vi "Write Standad Header Python.vi"(8 "error in (no error)":errorcluster, 11 "Save Image in":refnum<class "Save Image.lvclass">) -> (0 "error out":errorcluster, 3 "Save Image out":refnum<class "Save Image.lvclass">)   [LabVIEW 2018, in "Save Image.lvclass"]
uses:
  Save Image.lvclass
  Save Image.lvclass/Save Image.ctl
  Simulated_Header/Simulated_Header.lvclass
  Python Toolkit/Python Toolkit.lvclass
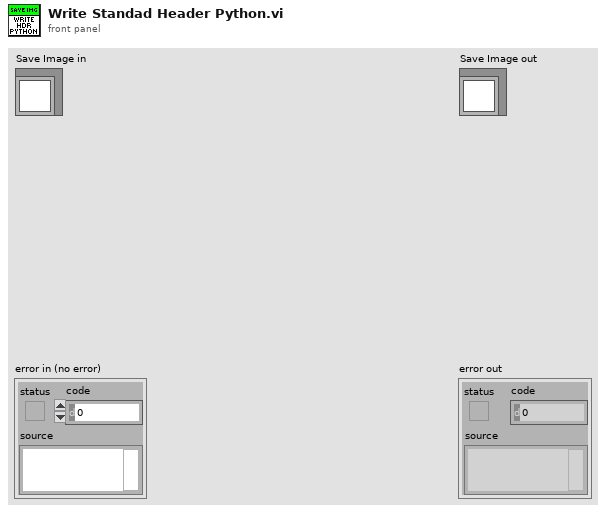
[diagram p1: front panel]
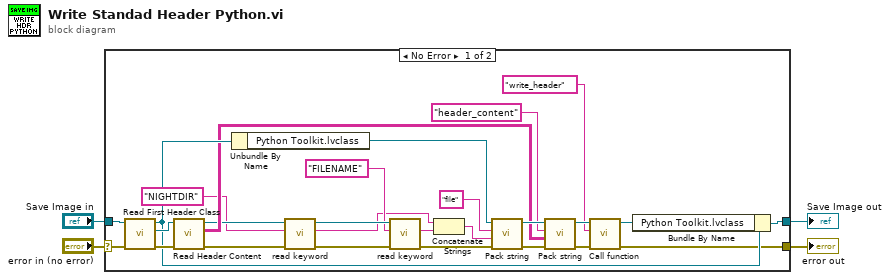
[diagram p0: block diagram]
diagram:
  n1 = case shown="No Error" "error in (no error)" {
    selector: "error in (no error)" -> [w31 w32]
    tunnel: [w24 w32] -> w1
    tunnel: [w26 w33] -> w2
    tunnel: "Save Image in" -> [w30 w33]
    frame No Error {
      n2 = call "Read First Header Class.vi"("error in (no error)"=w31, "Save Image in"=w30) -> ("error out"=w28:errorcluster, "Simulated_Header.lvclass"=w29:refnum<class "Simulated_Header.lvclass">, "Save Image out"=w27:refnum<class "Save Image.lvclass">)  [unwired: 7 in]
      n3 = call "Read Header Content.vi"("error in (no error)"=w28, "Simulated_Header in"=w29) -> ("error out"=w14:errorcluster, "Header Content"=w16:string[][], "Simulated_Header out"=w13:refnum<class "Simulated_Header.lvclass">)  [unwired: 7 in]
      n4 = Unbundle By Name(w27) -> ("Python Toolkit.lvclass"=w23:refnum<class "Python Toolkit.lvclass">)
      n5 = call "read keyword.vi"("error in (no error)"=w14, "keyword"="NIGHTDIR" ("Keyword Name"), "Simulated_Header in"=w13) -> ("error out"=w12:errorcluster, "value"=w6:string, "Simulated_Header out"=w11:refnum<class "Simulated_Header.lvclass">)  [unwired: 6 in]
      n6 = call "read keyword.vi"("error in (no error)"=w12, "keyword"="FILENAME" ("Keyword Name"), "Simulated_Header in"=w11) -> ("error out"=w8:errorcluster, "value"=w5:string)  [unwired: 6 in, 1 out]
      n7 = Concatenate Strings(w6, w5) -> (w7:string)
      n8 = call "Pack string.vi"("error in (no error)"=w8, "Argument"=w7, "Keyword Name"="file", "Python Toolkit in"=w23) -> ("error out"=w19:errorcluster, "Python Toolkit out"=w20:refnum<class "Python Toolkit.lvclass">)  [unwired: 6 in]
      n9 = call "Pack string.vi"("error in (no error)"=w19, "Argument"=w16, "Keyword Name"="header_content", "Python Toolkit in"=w20) -> ("error out"=w22:errorcluster, "Python Toolkit out"=w21:refnum<class "Python Toolkit.lvclass">)  [unwired: 6 in]
      n10 = call "Call function.vi"("error in (no error)"=w22, "Function Name"="write_header", "Python Toolkit in"=w21) -> ("error out"=w24:errorcluster, "Python Toolkit out"=w25:refnum<class "Python Toolkit.lvclass">)  [unwired: 7 in]
      n11 = Bundle By Name(cluster=w27, "Python Toolkit.lvclass"=w25) -> (w26:refnum<class "Save Image.lvclass">)
    }
    frame Error {
    }
  }
  "error out" <- w1
  "Save Image out" <- w2
